vi "Gather Mean.vi"(10 "JSON Statistics":refnum<class "JSON Running Mean.lvclass">, 11 "JSON Value In":refnum<class "JSON Value.lvclass">) -> (3 "JSON Statistic or Object":refnum<class "JSON Value.lvclass">)   [LabVIEW 2020, in "Library Commun.lvlib" / "JSON Running Mean.lvclass"]
uses:
  JSON Running Mean.lvclass
  JSON Value/JSON Value.lvclass
  C:/Users/ngarcin/OneDrive - Altyor/Standard TB/Class/JSON API/JSON Value/JSON Value.lvclass
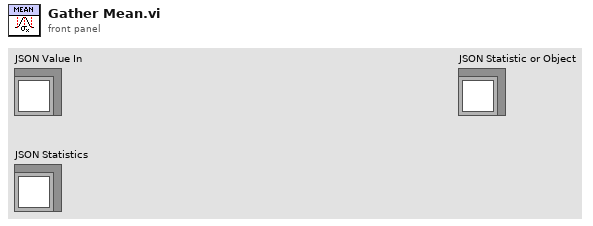
[diagram p1: front panel]
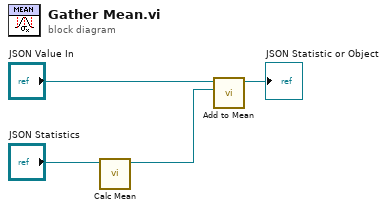
[diagram p0: block diagram]
diagram:
  n1 = call-dynamic "Calc Mean.vi"("JSON Statistics in"="JSON Statistics") -> ("JSON Value"=w1:refnum<class "JSON Value.lvclass">)  [unwired: 10 in]
  n2 = call-dynamic "Add to Mean.vi"("Non Object"=w1, "JSON Value In"="JSON Value In") -> ("JSON Mean out"=→"JSON Statistic or Object":refnum<class "JSON Running Mean.lvclass">)  [unwired: 9 in]
